vi "FPGA Add-On Specialty IO Example.vi"() -> ()   [LabVIEW 2017]
uses:
  Documents/github/NIVeristandAdd-ons/FPGA-Custom-Device/Source/FPGA/Speciality IO/Types/PWM.Measure.Digital.Measurement.ctl
  Documents/github/NIVeristandAdd-ons/FPGA-Custom-Device/Source/FPGA/Speciality IO/Types/PWM.Generate.Digital.Settings.ctl
  Documents/github/NIVeristandAdd-ons/FPGA-Custom-Device/Source/FPGA/Speciality IO/Types/PWM.Measure.Analog.Measurement.ctl
  Documents/github/NIVeristandAdd-ons/FPGA-Custom-Device/Source/FPGA/Speciality IO/Types/PWM.Measure.Digital.Settings.ctl
  Documents/github/NIVeristandAdd-ons/FPGA-Custom-Device/Source/FPGA/Speciality IO/Types/PWM.Measure.Analog.Settings.ctl
  Documents/github/NIVeristandAdd-ons/FPGA-Custom-Device/Source/FPGA/Speciality IO/Types/Sine.Generate.Settings.ctl
  <vilib>/Platform/TimedLoop/XDataNode/timing_clust.ctl
  <vilib>/Platform/TimedLoop/XDataNode/nitl_modes.ctl
  <vilib>/Platform/TimedLoop/XDataNode/wakeup.ctl
  <vilib>/rvi/Emulation/niFpgaGetClockAttributes.vi
  <vilib>/rvi/Emulation/niFpgaSctlEmulationGetInTimedLoop.vi
  <vilib>/rvi/Emulation/niFpgaEmulationReportErrorSimple.vi
  <vilib>/rvi/Emulation/niFpgaCriticalErrorInLSC.vi
  <vilib>/Platform/TimedLoop/XDataNode/XDataNode.xnode
  Documents/github/NIVeristandAdd-ons/FPGA-Custom-Device/Source/FPGA/Speciality IO/Speciality FPGA IO.lvlib
  <vilib>/Platform/TimedLoop/XDataNode/XDNodeRunTimeDep.lvlib
panel:
  out "Analog.Generation.Ticks":u32=10 caption="Count(uSec)"
  in  "Generate.Sine.Ch1.Settings":T1
  in  "Generate.Sine.Ch0.Settings":T1
  in  "Sine":bool=TRUE
  in  "Measure.Analog.Ch1.Settings":T2={"ACTIVE EDGE"=FALSE, "TIMEOUT"=40000000, "THRESHOLD"=95.0}
  in  "Measure.Analog.Ch0.Settings":T2={"ACTIVE EDGE"=TRUE, "TIMEOUT"=40000000, "THRESHOLD"=0.0}
  in  "Measure.Digital.Ch1.Settings":T3={"ACTIVE EDGE"=FALSE, "TIMEOUT"=40000000}
  in  "Measure.Digital.Ch0.Settings":T3={"ACTIVE EDGE"=TRUE, "TIMEOUT"=40000000}
  out "Measure.Analog.Ch1":T4={"ACTIVE TICKS"=90, "INACTIVE TICKS"=10, "ACQ TICKS"=400, "ACTIVE VOLTAGE"=-6.998723030090332, "INACTIVE VOLTAGE"=6.998509407043457}
  out "Measure.Analog.Ch0":T4={"ACTIVE TICKS"=10, "INACTIVE TICKS"=10, "ACQ TICKS"=400, "ACTIVE VOLTAGE"=4.979251861572266, "INACTIVE VOLTAGE"=-4.979404449462891}
  in  "Generate.Digital.Ch1.Internal.Settings":T5={"ACTIVE EDGE"=FALSE, "ACTIVE TICKS"=60000000, "INACTIVE TICKS"=20000000}
  in  "Generate.Digital.Ch0.Internal.Settings":T5={"ACTIVE EDGE"=TRUE, "ACTIVE TICKS"=4000, "INACTIVE TICKS"=12000}
  out "Measure.Digital.Ch1":T6
  out "Measure.Digital.Ch0":T6={"ACTIVE TICKS"=4000, "INACTIVE TICKS"=12000, "ACQ TICKS"=1}
  in  "Analog.Generation.Ticks":u32=10 caption="Count(uSec)"
  # "98"
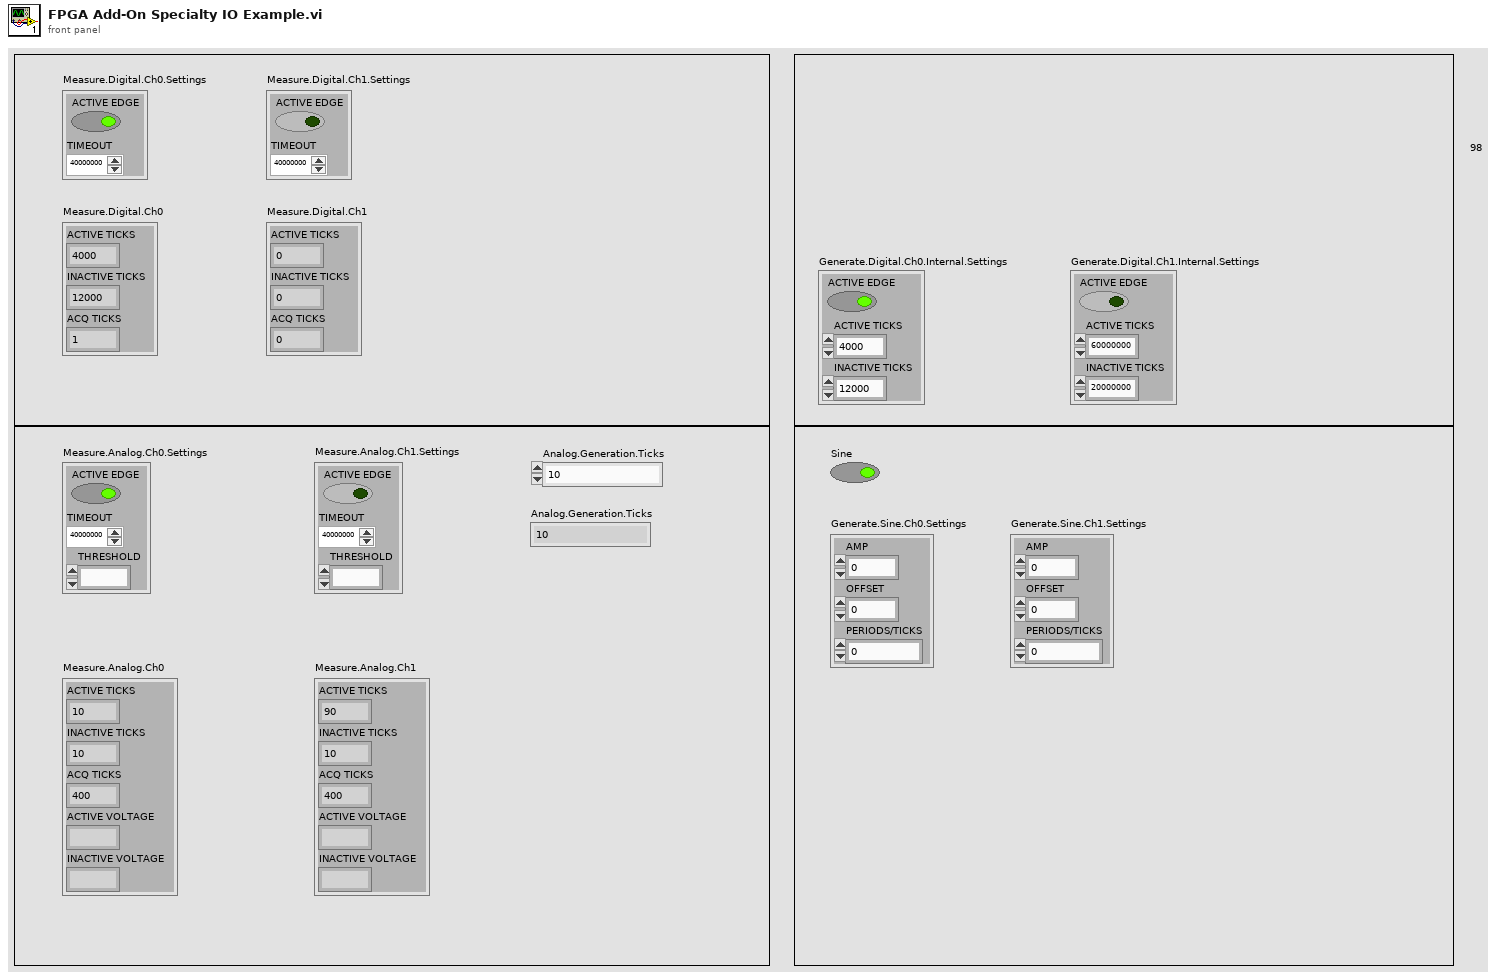
[diagram p1: front panel]
types:
  T1 = typedef "Speciality FPGA IO.lvlib/Sine.Generate.Settings.ctl" = cluster{"AMP":fxp<+/-,32,8>, "OFFSET":fxp<+/-,32,8>, "PERIODS/TICKS":fxp<+,32,0>}
  T2 = typedef "Speciality FPGA IO.lvlib/PWM.Measure.Analog.Settings.ctl" = cluster{"ACTIVE EDGE":bool, "TIMEOUT":u32, "THRESHOLD":fxp<+/-,32,8>}
  T3 = typedef "Speciality FPGA IO.lvlib/PWM.Measure.Digital.Settings.ctl" = cluster{"ACTIVE EDGE":bool, "TIMEOUT":u32}
  T4 = typedef "Speciality FPGA IO.lvlib/PWM.Measure.Analog.Measurement.ctl" = cluster{"ACTIVE TICKS":u32, "INACTIVE TICKS":u32, "ACQ TICKS":u32, "ACTIVE VOLTAGE":fxp<+/-,32,8>, "INACTIVE VOLTAGE":fxp<+/-,32,8>}
  T5 = typedef "Speciality FPGA IO.lvlib/PWM.Generate.Digital.Settings.ctl" = cluster{"ACTIVE EDGE":bool, "ACTIVE TICKS":u32, "INACTIVE TICKS":u32}
  T6 = typedef "Speciality FPGA IO.lvlib/PWM.Measure.Digital.Measurement.ctl" = cluster{"ACTIVE TICKS":u32, "INACTIVE TICKS":u32, "ACQ TICKS":u32}
  T7 = typedef "XDNodeRunTimeDep.lvlib/timing_clust.ctl" = cluster{"Expected End [f-1]":u64, "Actual End [f-1]":u64, "Finished Late? [f-1]":bool, "Expected End [i-1]":u64, "Actual End [i-1]":u64, "Finished Late? [i-1]":bool, "Expected Start [i]":u64, "Actual Start [i]":u64, "Expected Start [f]":u64, "Actual Start [f]":u64, "Source Name":string, "Structure Name":string, "Period":i64, "Deadline":i64, "Offset":i64, "Start":i64, "Priority":i32, "Timeout":i32, "Mode":T8, "Wakeup Reason":T9, "Error":errorcluster, "Source Type":string, "Secondary Source Type":string, "Global End Time":u64, "Global Start Time":u64, "Frame Duration":u64, "Iteration Duration":u64, "Assigned CPU":i32, "I/O Scan Engine Mode":u32}
  T8 = typedef "XDNodeRunTimeDep.lvlib/nitl_modes.ctl" = enum32{"No Change", "Process missed periods, maintain original phase", "Discard missed periods, maintain original phase", "Process missed periods, ignore original phase", "Discard missed periods, ignore original phase"}
  T9 = typedef "XDNodeRunTimeDep.lvlib/wakeup.ctl" = enum32{"Normal", "Aborted", "Asynchronous wakeup", "Timing source error", "Timed loop error", "Timeout"}
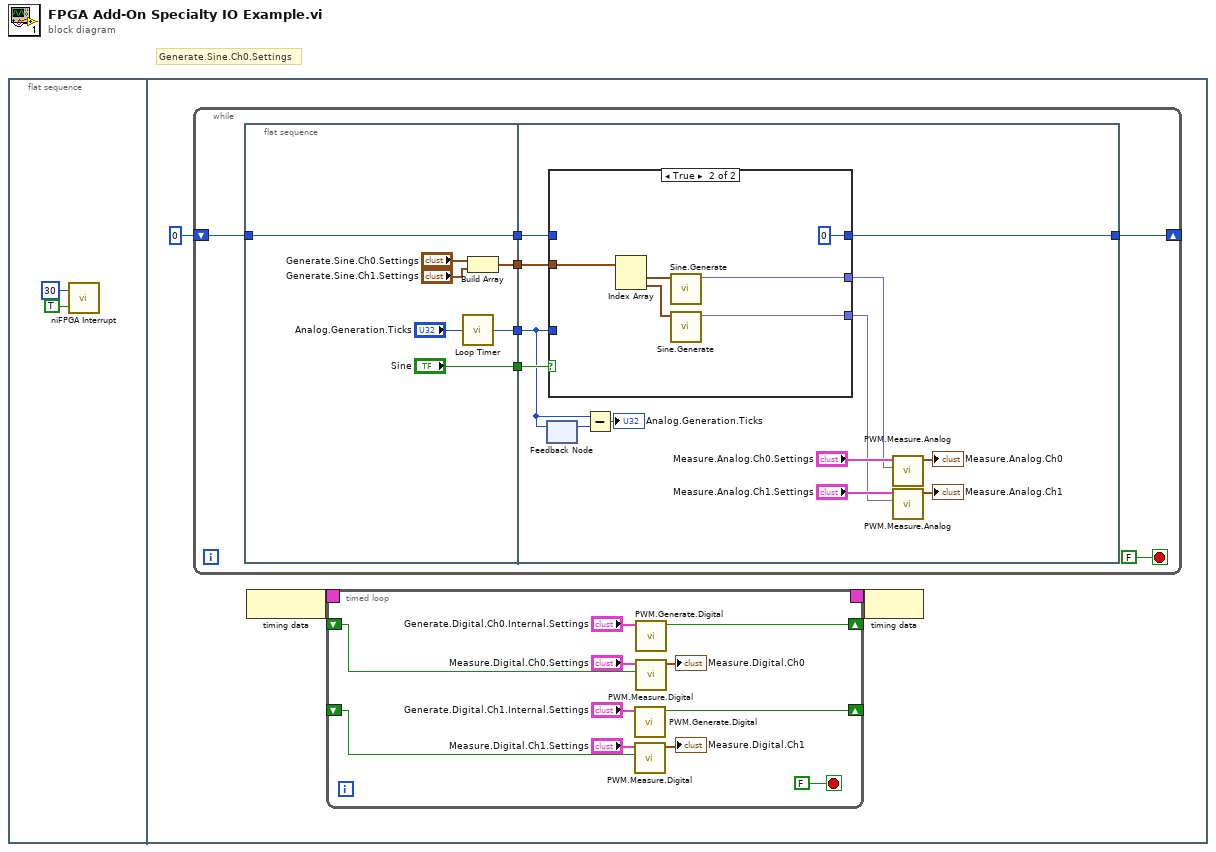
[diagram p0: block diagram]
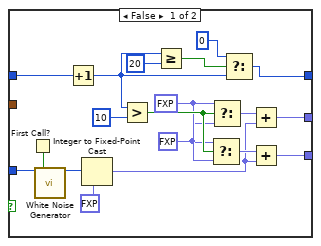
[diagram p2: hidden frame]
diagram:
  # "Generate.Sine.Ch0.Settings"
  n1 = flat-sequence {
    frame #0 {
      n2 = call <vilib>:"niFPGA Interrupt.vi"("Wait Until Cleared (F)"=TRUE, "IRQ Number (0)"=u8 30) -> ()  [unwired: 1 in]
    }
    frame #1 {
      n3 = while {
        shift-right: [w25] -> _
        shift-left: i16 0 -> [w26]
        stop <- FALSE stop-if-true
        n4 = flat-sequence {
          tunnel: [w33] -> w27
          tunnel: w26 -> [w33]
          tunnel: [w32] -> w24
          tunnel: ["Sine"] -> w22
          tunnel: [w28] -> w21
          tunnel: w27 -> [w40]
          tunnel: [w41] -> w25
          tunnel: w24 -> [w36]
          tunnel: w22 -> [w39]
          tunnel: w21 -> [w38]
          frame #0 {
            n5 = call "Loop Timer"("Count(uSec)"="Analog.Generation.Ticks") -> ("Tick Count(uSec)"=w32:u32)
            n6 = Build Array("Generate.Sine.Ch0.Settings", "Generate.Sine.Ch1.Settings") -> (w28:T1[])
          }
          frame #1 {
            n7 = feedback-in #1(w36) -> ()
            n8 = feedback #1() -> (w37:u32)  [unwired: 1 in]
            n9 = case shown="True" w39 {
              tunnel: [w49 w67] -> w43
              tunnel: [w50 w68] -> w42
              tunnel: w40 -> [w53 _]
              tunnel: w36 -> [w52 _]
              tunnel: [w51 i16 0 ("t")] -> w41
              tunnel: w38 -> [_ w71]
              frame False {
                w60 = fxp<+/-,32,8> 12.0 ("t")
                w61 = fxp<+/-,32,8> -12.0 ("PWM")
                n10 = First Call?() -> (First Call?: T/F=w59:bool)
                n11 = call "White Noise Generator"("seed"=w52, "reset"=w59) -> ("white noise out"=w58:i16)  [unwired: 13 in]
                n12 = Increment(x=w53) -> (x+1=w63:i16)
                n13 = Integer to Fixed-Point Cast(fixed-point type=fxp<+/-,16,1> 0.0, integer=w58) -> (fixed-point=w48:fxp<+/-,16,1>)
                n14 = Greater?(x=w63, y=i16 10) -> (0:w62:bool)
                n15 = Greater Or Equal?(x=w63, y=i16 20) -> (x >= y?=w54:bool)
                n16 = Select(t=w60, s=w62, f=w61) -> (s? t:f=w55:fxp<+/-,32,8>)
                n17 = Select(t=w61, s=w62, f=w60) -> (s? t:f=w56:fxp<+/-,32,8>)
                n18 = Select(t=i16 0, s=w54, f=w63) -> (s? t:f=w51:i16)
                n19 = Add(x=w56, y=w48) -> (x+y=w50:fxp<+/-,33,9>)
                n20 = Add(x=w55, y=w48) -> (x+y=w49:fxp<+/-,33,9>)
              }
              frame True {
                n21 = Index Array(array=w71) -> (element #1=w70:T1, element #2=w69:T1)  [unwired: 2 in]
                n22 = call "Sine.Generate.vi"("Settings"=w70) -> ("Output"=w68:fxp<+/-,32,8>)  [unwired: 10 in]
                n23 = call "Sine.Generate.vi"("Settings"=w69) -> ("Output"=w67:fxp<+/-,32,8>)  [unwired: 10 in]
              }
            }
            n24 = Subtract(x=w36, y=w37) -> (x-y=→"Analog.Generation.Ticks":u32)
            n25 = call "PWM.Measure.Analog.vi"("PWM"=w42, "Settings"="Measure.Analog.Ch0.Settings") -> ("Measurement"=→"Measure.Analog.Ch0":T4)  [unwired: 8 in, 1 out]
            n26 = call "PWM.Measure.Analog.vi"("PWM"=w43, "Settings"="Measure.Analog.Ch1.Settings") -> ("Measurement"=→"Measure.Analog.Ch1":T4)  [unwired: 8 in, 1 out]
          }
        }
      }
      n27 = node-c288() -> (w5:T7)
      n28 = timed-loop {
        timing: w5 -> [_]
        timing-out: [_] -> w4
        shift-right: [w15] -> _
        shift-left: _ -> [w14]
        shift-right: [w13] -> _
        shift-left: _ -> [w12]
        stop <- FALSE stop-if-true
        n29 = call "PWM.Generate.Digital.vi"("Settings"="Generate.Digital.Ch1.Internal.Settings") -> ("Output"=w15:bool)  [unwired: 10 in]
        n30 = call "PWM.Measure.Digital.vi"("State"=w14, "Settings"="Measure.Digital.Ch1.Settings") -> ("Measurement"=→"Measure.Digital.Ch1":T6)  [unwired: 8 in, 1 out]
        n31 = call "PWM.Generate.Digital.vi"("Settings"="Generate.Digital.Ch0.Internal.Settings") -> ("Output"=w13:bool)  [unwired: 10 in]
        n32 = call "PWM.Measure.Digital.vi"("State"=w12, "Settings"="Measure.Digital.Ch0.Settings") -> ("Measurement"=→"Measure.Digital.Ch0":T6)  [unwired: 8 in, 1 out]
      }
      n33 = node-c288(w4) -> ()
    }
  }
